vi "Untitled 4.vi"   [LabVIEW 2015]
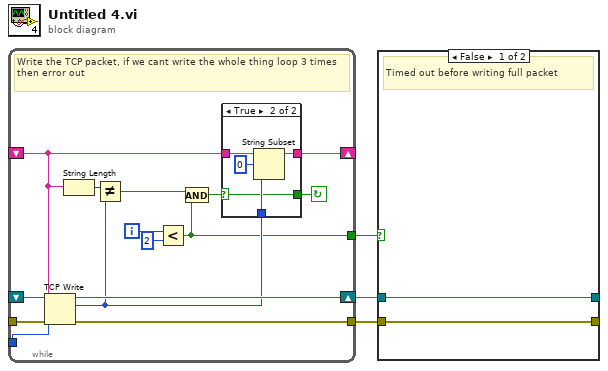
[diagram p0: block diagram]
diagram:
  n1 = while {
    tunnel: _ -> [w15]
    shift-right: [w18] -> w2
    shift-left: _ -> [w16]
    shift-right: [w13] -> _
    shift-left: _ -> [w11]
    tunnel: _ -> [w14]
    tunnel: [w17] -> w3
    tunnel: [w4] -> w1
    i -> [w8]
    stop <- w12 continue-if-true
    # "Write the TCP packet, if we cant write the whole thing loop 3 times then error out"
    n2 = TCP Write(connection ID=w16, data in=w11, error in (no error)=w14, 9:w15) -> (connection ID out=w18:refnum<k5>, bytes written=w9:i32, error out=w17:errorcluster)
    n3 = String Length(string=w11) -> (length=w10:i32)
    n4 = Not Equal?(x=w10, y=w9) -> (x != y?=w6:bool)
    n5 = Less?(x=w8, y=2) -> (x < y?=w4:bool)
    n6 = And(x=w6, y=w4) -> (x .and. y?=w5:bool)
    n7 = case shown="True" w5 {
      selector: w5 -> [w19 w21]
      tunnel: [w20 w22] -> w13
      tunnel: w11 -> [w20 w23]
      tunnel: [w19 w21] -> w12
      tunnel: w9 -> [_ w24]
      frame False {
      }
      frame True {
        n8 = String Subset(string=w23, offset (0)=0, length (rest)=w24) -> (substring=w22:string)
      }
    }
  }
  n9 = case shown="False" w1 {
    tunnel: w3 -> [w26 w28]
    tunnel: [w27 w29] -> _
    tunnel: w2 -> [w27 w29]
    tunnel: [w26 w28] -> _
    frame False {
      # "Timed out before writing full packet"
    }
    frame True {
      # "everything was written"
    }
  }
